vi "execute.vi"(8 "error in (no error)":errorcluster, 10 "Context in":refnum<class "Context.lvclass">, 11 "ApplyAOSCorrectionByForcesCommand in":refnum<class "ApplyAOSCorrectionByForcesCommand.lvclass">) -> (0 "error out":errorcluster, 2 "Context out":refnum<class "Context.lvclass">, 3 "ApplyAOSCorrectionByForcesCommand out":refnum<class "ApplyAOSCorrectionByForcesCommand.lvclass">)   [LabVIEW 2016, in "ApplyAOSCorrectionByForcesCommand.lvclass"]
uses:
  ApplyAOSCorrectionByForcesCommand.lvclass
  Context/Context.lvclass
  ApplyAOSCorrectionByForcesCommand.lvclass/ApplyAOSCorrectionByForcesCommand.ctl
  Context/Context.lvclass/Context.ctl
  Context/getModel.vi
  Context/setModel.vi
  Model/getState.vi
  States/State/State.lvclass
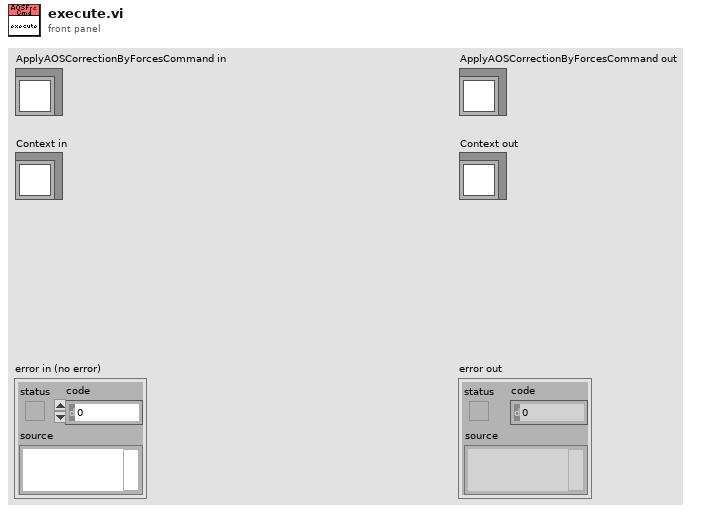
[diagram p1: front panel]
types:
  T1 = typedef "M1M3SupportTopics.lvlib/CommandApplyAOSCorrectionByForces.ctl" = cluster{"CommandId":T2, "ZForces":dbl[]}
  T2 = typedef "M1M3SupportTopics.lvlib/CommandId.ctl" = i32
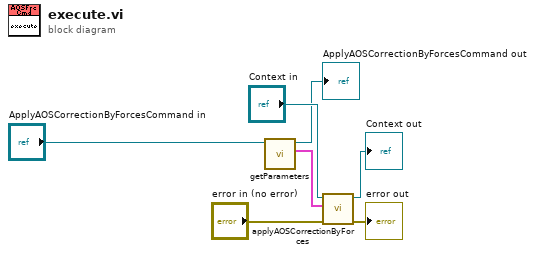
[diagram p0: block diagram]
diagram:
  n1 = call "getParameters.vi"("ApplyAOSCorrectionByForcesCommand in"="ApplyAOSCorrectionByForcesCommand in") -> ("Parameters"=w6:T1, "ApplyAOSCorrectionByForcesCommand out"=→"ApplyAOSCorrectionByForcesCommand out":refnum<class "ApplyAOSCorrectionByForcesCommand.lvclass">)  [unwired: 9 in]
  n2 = call "applyAOSCorrectionByForces.vi"("error in (no error)"="error in (no error)", "Parameters"=w6, "Context in"="Context in") -> ("error out"=→"error out":errorcluster, "Context out"=→"Context out":refnum<class "Context.lvclass">)  [unwired: 7 in]
